vi "LINE1.vi"(0 "Frequency(Hz)":i32, 1 "LOL(V)":dbl, 2 "HIL(V)":dbl, 3 "Laser GPIB":u8=10 max=100, 4 "Enable time(ms)":u32, 5 "DTY":i32, 6 "t_before(ms)":u32, 7 "Current (mA)":dbl, 8 "y-dist":i32, 9 "x-dist":i32, 10 "speed":u16, 11 "Motor GPIB":u8=6) -> ()   [LabVIEW 2010]
uses:
  <vilib>/express/express arith-compare/Formula/XNode/ExpressFormulaBlockNode.xnode
panel:
  out "resulting string":string
  out "Dummy":string
  # "LINE1<space>[Displacement]<space>[Speed]<space>[Current]<space>[wait]<space>[repetitions]"
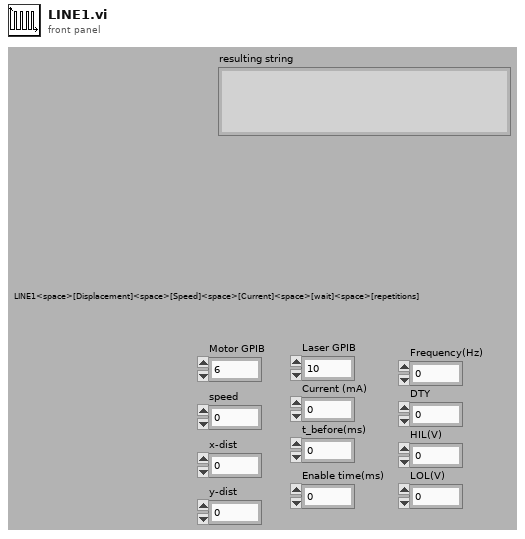
[diagram p1: front panel]
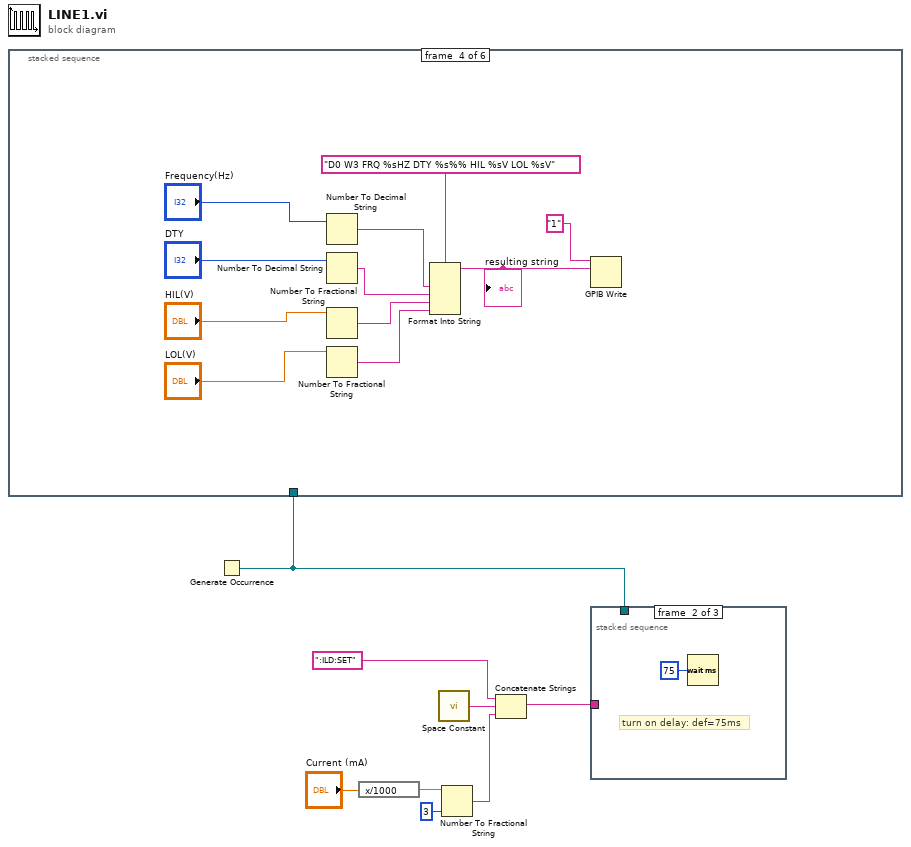
[diagram p0: block diagram]
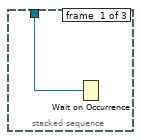
[diagram p2: hidden frame]
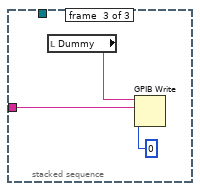
[diagram p3: hidden frame]
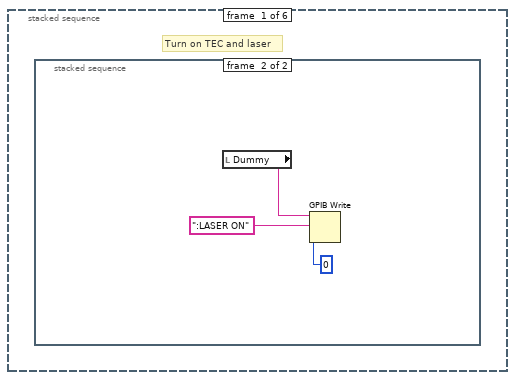
[diagram p4: hidden frame]
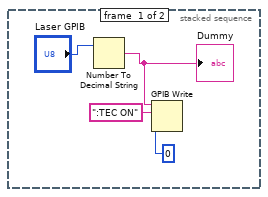
[diagram p5: hidden frame]
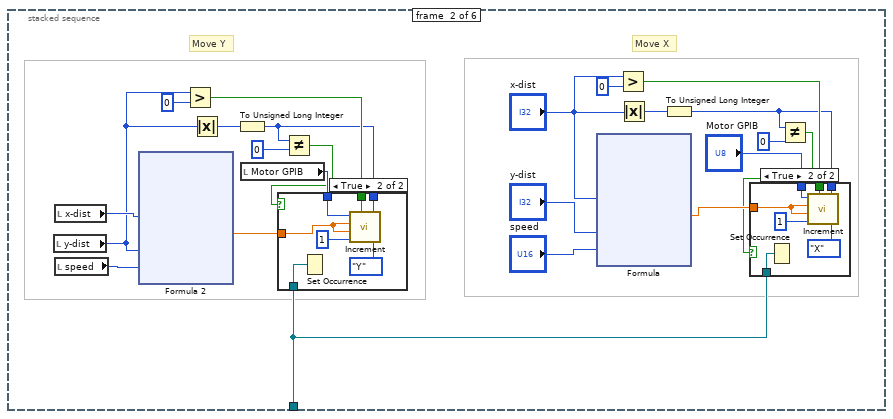
[diagram p6: hidden frame]
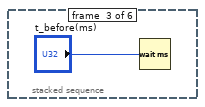
[diagram p9: hidden frame]
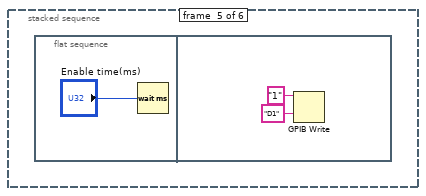
[diagram p10: hidden frame]
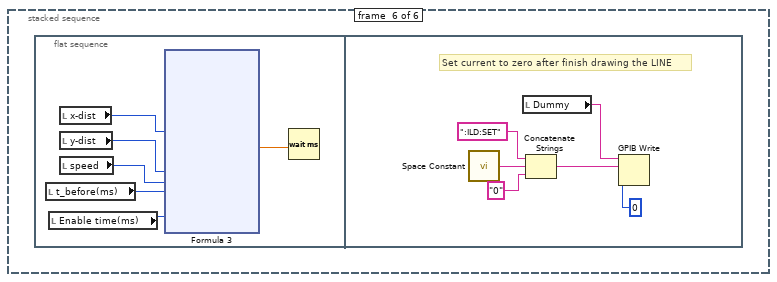
[diagram p11: hidden frame]
diagram:
  n1 = Generate Occurrence() -> (w1:refnum<k4>)
  n2 = stacked-sequence {
    tunnel: w1 -> [_ w16 _ _ _ _]
    frame #0 {
      # "Turn on TEC and laser"
      n3 = stacked-sequence {
        frame #0 {
          n4 = Number To Decimal String(number="Laser GPIB") -> (decimal integer string=w10:string)  [unwired: 1 in]
          "Dummy" <- w10
          n5 = GPIB Write(0:w10, 1:":TEC ON" ("data"), 2:i16 0 ("mode (0)")) -> ()  [unwired: 2 in, 2 out]
        }
        frame #1 {
          n6 = local read "Dummy"() -> (w14:string)
          n7 = GPIB Write(0:w14, 1:":LASER ON" ("data"), 2:i16 0 ("mode (0)")) -> ()  [unwired: 2 in, 2 out]
        }
      }
    }
    frame #1 {
      # "Move X"
      # "Move Y"
      n8 = local read "y-dist"() -> (w32:i32)
      n9 = local read "x-dist"() -> (w34:i32)
      n10 = local read "speed"() -> (w38:u16)
      n11 = xnode "Formula 2"("X1"=w34, "X2"=w32, "X3"=w38) -> ("Result"=w24:dbl)  [unwired: 1 in, 1 out]
      n12 = Greater?(x=w32, y=0) -> (0:w35:bool)
      n13 = Absolute Value(x=w32) -> (abs(x)=w33:i32)
      n14 = To Unsigned Long Integer(number=w33) -> (unsigned 32bit integer=w22:u32)
      n15 = local read "Motor GPIB"() -> (w37:u8)
      n16 = Not Equal?(x=w22, y=u32 0) -> (x != y?=w20:bool)
      n17 = case shown="True" w20 {
        tunnel: w37 -> [_ w50]
        tunnel: w35 -> [_ w49]
        tunnel: w22 -> [_ w48]
        tunnel: w24 -> [_ w47]
        tunnel: w16 -> [_ w46]
        frame False {
        }
        frame True {
          n18 = Set Occurrence(w46) -> ()
          n19 = call "Increment.vi"("GPIB_Addr"=w50, "F Speed"=w47, "L Speed"=w47, "Rate"=u16 1, "CCW 3"=w49, "Distance"=w48, "Axis"=enum16{"X", "Y", "Z", "U", "V", "W"}."Y") -> ()
        }
      }
      n20 = xnode "Formula"("X1"="x-dist", "X2"="y-dist", "X3"="speed") -> ("Result"=w23:dbl)  [unwired: 1 in, 1 out]
      n21 = Greater?(x="x-dist", y=0) -> (0:w28:bool)
      n22 = Absolute Value(x="x-dist") -> (abs(x)=w25:i32)
      n23 = To Unsigned Long Integer(number=w25) -> (unsigned 32bit integer=w19:u32)
      n24 = Not Equal?(x=w19, y=u32 0) -> (x != y?=w17:bool)
      n25 = case shown="True" w17 {
        tunnel: "Motor GPIB" -> [_ w45]
        tunnel: w28 -> [_ w42]
        tunnel: w19 -> [_ w41]
        tunnel: w23 -> [_ w40]
        tunnel: w16 -> [_ w39]
        frame False {
        }
        frame True {
          n26 = Set Occurrence(w39) -> ()
          n27 = call "Increment.vi"("GPIB_Addr"=w45, "F Speed"=w40, "L Speed"=w40, "Rate"=u16 1, "CCW 3"=w42, "Distance"=w41, "Axis"=enum16{"X", "Y", "Z", "U", "V", "W"}."X") -> ()
        }
      }
    }
    frame #2 {
      n28 = Wait (ms)(milliseconds to wait="t_before(ms)") -> ()  [unwired: 1 out]
    }
    frame #3 {
      n29 = Number To Decimal String(number="Frequency(Hz)") -> (decimal integer string=w81:string)  [unwired: 1 in]
      n30 = Number To Decimal String(number="DTY") -> (decimal integer string=w80:string)  [unwired: 1 in]
      n31 = Number To Fractional String(number="HIL(V)") -> (F-format string=w83:string)  [unwired: 3 in]
      n32 = Number To Fractional String(number="LOL(V)") -> (F-format string=w85:string)  [unwired: 3 in]
      n33 = Format Into String(format string="D0 W3 FRQ %sHZ DTY %s%% HIL %sV LOL %sV", w81, w80, w83, w85) -> (resulting string=w88:string)  [unwired: 2 in, 1 out]
      "resulting string" <- w88
      n34 = GPIB Write(0:"1" ("address string"), 1:w88) -> ()  [unwired: 3 in, 2 out]
    }
    frame #4 {
      n35 = flat-sequence {
        frame #0 {
          n36 = Wait (ms)(milliseconds to wait="Enable time(ms)") -> ()  [unwired: 1 out]
        }
        frame #1 {
          n37 = GPIB Write(0:"1" ("address string"), 1:"D1" ("data")) -> ()  [unwired: 3 in, 2 out]
        }
      }
    }
    frame #5 {
      n38 = flat-sequence {
        frame #0 {
          n39 = local read "t_before(ms)"() -> (w93:u32)
          n40 = local read "Enable time(ms)"() -> (w92:u32)
          n41 = local read "x-dist"() -> (w96:i32)
          n42 = local read "y-dist"() -> (w95:i32)
          n43 = local read "speed"() -> (w94:u16)
          n44 = xnode "Formula 3"("X1"=w96, "X2"=w95, "X3"=w94, "X4"=w93, "X5"=w92) -> ("Result"=w97:dbl)  [unwired: 1 in, 1 out]
          n45 = Wait (ms)(milliseconds to wait=w97) -> ()  [unwired: 1 out]
        }
        frame #1 {
          # "Set current to zero after finish drawing the LINE"
          n46 = call <vilib>:"Space Constant.vi"() -> ("String"=w117:string)
          n47 = local read "Dummy"() -> (w114:string)
          n48 = Concatenate Strings(":ILD:SET", w117, "0" ("string")) -> (w116:string)
          n49 = GPIB Write(0:w114, 1:w116, 2:i16 0 ("mode (0)")) -> ()  [unwired: 2 in, 2 out]
        }
      }
    }
  }
  n50 = expression code="x/1000"("Current (mA)") -> (w2:dbl)
  n51 = call <vilib>:"Space Constant.vi"() -> ("String"=w7:string)
  n52 = Number To Fractional String(number=w2, precision (6)=i16 3) -> (F-format string=w5:string)  [unwired: 2 in]
  n53 = Concatenate Strings(":ILD:SET", w7, w5) -> (w8:string)
  n54 = stacked-sequence {
    tunnel: w8 -> [_ _ w123]
    tunnel: w1 -> [w120 _ _]
    frame #0 {
      n55 = Wait on Occurrence(2:w120) -> ()  [unwired: 2 in, 1 out]
    }
    frame #1 {
      # "turn on delay: def=75ms"
      n56 = Wait (ms)(milliseconds to wait=u32 75) -> ()  [unwired: 1 out]
    }
    frame #2 {
      n57 = local read "Dummy"() -> (w124:string)
      n58 = GPIB Write(0:w124, 1:w123, 2:i16 0 ("mode (0)")) -> ()  [unwired: 2 in, 2 out]
    }
  }
